vi "GetEvtReports.vi"(8 "error in (no error)":errorcluster, 11 "UserEvtPlugins in":refnum<class "UserEvtPlugins.lvclass">) -> (0 "error out":errorcluster, 3 "UserEvtPlugins out":refnum<class "UserEvtPlugins.lvclass">)   [LabVIEW 2014, in "EventPlugins.lvlib" / "UserEvtPlugins.lvclass"]
uses:
  UserEvtPlugins.lvclass
  <userlib>/NIST/BaseClasses/BasePlugin_class/BasePlugin.lvclass/BasePlugin.ctl
  EventPluginBaseClass/EventPluginBaseClass.lvclass/EventPluginBaseClass.ctl
  EventPluginBaseClass/TypeDefs/clEvtReport.ctl
  <userlib>/NIST/BaseClasses/BasePlugin_class/Accessors/Read PluginIniFilePath.vi
  EventPluginBaseClass/Accessors/Read BusNumber.vi
  EventPluginBaseClass/Accessors/Read TimeArray.vi
  EventPluginBaseClass/Accessors/Read EvtParams.vi
  EventPluginBaseClass/Accessors/Read EvtConfig.vi
  <vilib>/Utility/config.llb/Read Key (String).vi
  <vilib>/Utility/config.llb/NI_LVConfig.lvlib
  EventPluginBaseClass/EventPluginBaseClass.lvclass
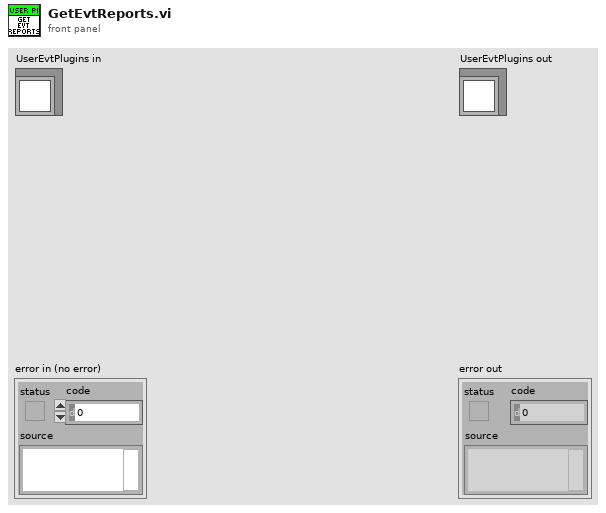
[diagram p1: front panel]
types:
  T1 = typedef "EventPlugins.lvlib/EventPluginBaseClass.lvclass/clEvtReport.ctl" = cluster{"Timestamp":dbl, "Synx":cdb[], "Freq":dbl, "ROCOF":dbl, "ID":i16}
  T2 = typedef "EventPlugins.lvlib/EventPluginBaseClass.lvclass/clEvtConfig.ctl" = cluster{"T0(UTC)":dbl, "F0":dbl, "Fs":i32, "FSamp":u32, "bPosSeq":bool}
  T3 = typedef "NI_LVConfig.lvlib/Config Data RefNum.ctl" = refnum<k1>
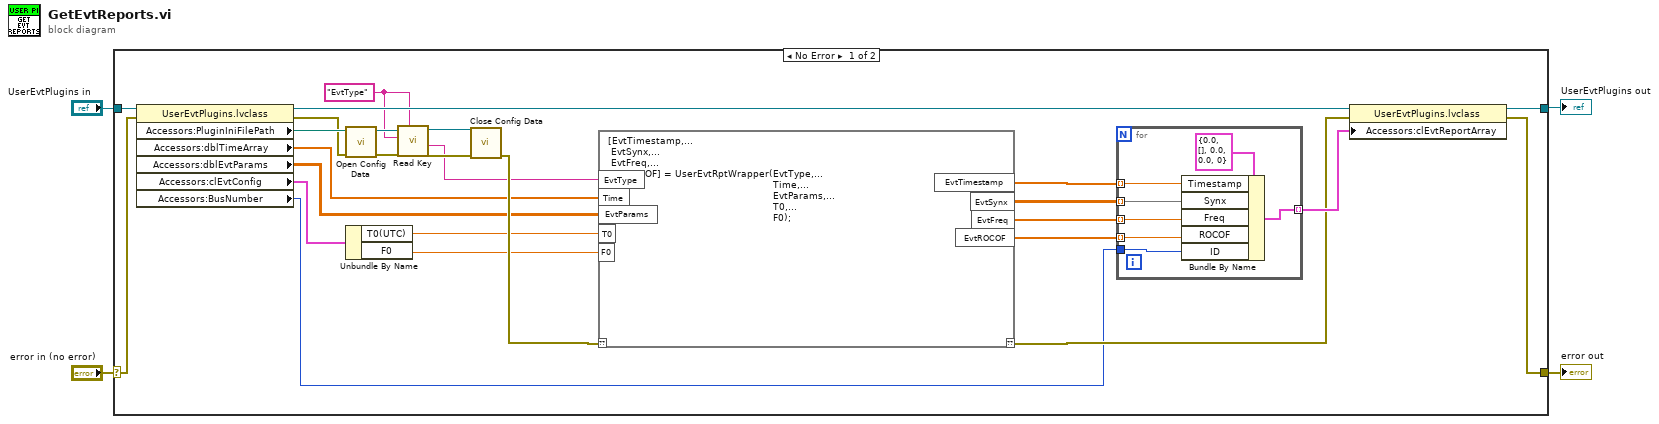
[diagram p0: block diagram]
diagram:
  n1 = case shown="No Error" "error in (no error)" {
    selector: "error in (no error)" -> [w28 w39]
    tunnel: [w12 w39] -> w1
    tunnel: [w13 w38] -> w2
    tunnel: "UserEvtPlugins in" -> [w30 w38]
    frame No Error {
      w23 = "EvtType" ("section")
      n2 = property class="UserEvtPlugins.lvclass"(reference=w30, error in=w28) -> (reference out=w29:refnum<class "UserEvtPlugins.lvclass">, error out=w26:errorcluster, "Accessors:PluginIniFilePath"=w27:path, "Accessors:dblTimeArray"=w18:dbl[], "Accessors:dblEvtParams"=w17:dbl[][], "Accessors:clEvtConfig"=w16:T2, "Accessors:BusNumber"=w5:u8)
      n3 = call <vilib>:"Open Config Data.vi"("error in (no error)"=w26, "configuration file path"=w27) -> ("error out"=w25:errorcluster, "refnum"=w24:T3)  [unwired: 7 in, 1 out]
      n4 = Unbundle By Name(w16) -> ("T0(UTC)"=w15:dbl, "F0"=w14:dbl)
      n5 = call-poly <vilib>:"Read Key.vi"("section"=w23, "error in (no error)"=w25, "key"=w23, "refnum"=w24) -> ("error out"=w21:errorcluster, "value"=w19:string, "refnum out"=w22:T3)  [unwired: 4 in, 1 out]
      n6 = call <vilib>:"Close Config Data.vi"("error in (no error)"=w21, "refnum"=w22) -> ("error out"=w20:errorcluster)  [unwired: 8 in, 1 out]
      n7 = script code="[EvtTimestamp,...\n EvtSynx,...\n EvtFreq,...\n EvtROCOF] = UserEvtRptWrapper(EvtType,...\n                                                       Time,...\n                                                       EvtParams,...\n                                                       T0,...\n                                                       F0);"("??"=w20, "EvtType"=w19, "Time"=w18, "EvtParams"=w17, "T0"=w15, "F0"=w14) -> ("??"=w6:errorcluster, "EvtTimestamp"=w11:dbl[], "EvtSynx"=w10:cdb[][], "EvtFreq"=w9:dbl[], "EvtROCOF"=w8:dbl[])
      n8 = for {
        tunnel: w11 -> [w36] mode=indexing
        tunnel: w10 -> [w35] mode=indexing
        tunnel: w9 -> [w34] mode=indexing
        tunnel: w8 -> [w33] mode=indexing
        tunnel: [w32] -> w7 mode=indexing
        tunnel: w5 -> [w31]
        n9 = Bundle By Name(cluster=T1 {"Timestamp"=0.0, "Synx"=[], "Freq"=0.0, "ROCOF"=0.0, "ID"=0} ("clEvtReport"), "Timestamp"=w36, "Synx"=w35, "Freq"=w34, "ROCOF"=w33, "ID"=w31) -> (w32:T1)
      }
      n10 = property class="UserEvtPlugins.lvclass"(reference=w29, error in=w6, "Accessors:clEvtReportArray"=w7) -> (reference out=w13:refnum<class "UserEvtPlugins.lvclass">, error out=w12:errorcluster)
    }
    frame Error {
    }
  }
  "error out" <- w1
  "UserEvtPlugins out" <- w2
